vi "mclb_move_and_resize.vi"(8 "error in (no error)":errorcluster, 10 "Panel Resize.NewBnds":T3, 11 "mclb in":refnum<vi>) -> (0 "error out":errorcluster, 1 "MCLB.Bounds":T2, 2 "MCLB.Position":T1, 3 "mclb out":refnum<vi>, 4 "FP.Height":u32)   [LabVIEW 2017, in "rywindow.lvclass"]
uses:
  rywindow.lvclass
  <vilib>/Utility/miscctls.llb/LVRectTypeDef.ctl
  <vilib>/Utility/miscctls.llb/LVBoundsTypeDef.ctl
  <vilib>/Utility/miscctls.llb/LVPositionTypeDef.ctl
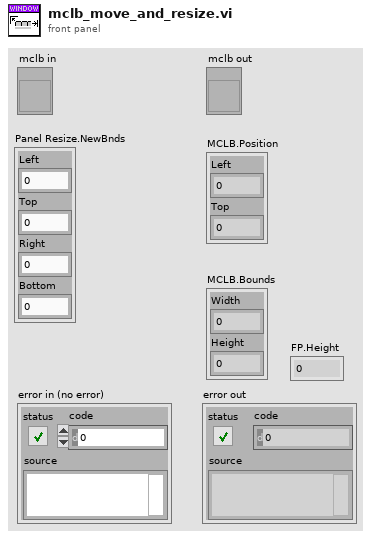
[diagram p1: front panel]
types:
  T1 = typedef "LVPositionTypeDef.ctl" = cluster{"Left":i32, "Top":i32}
  T2 = typedef "LVBoundsTypeDef.ctl" = cluster{"Width":u32, "Height":u32}
  T3 = typedef "LVRectTypeDef.ctl" = cluster{"Left":i16, "Top":i16, "Right":i16, "Bottom":i16}
  T4 = typedef "LVPointTypeDef.ctl" = cluster{"Horizontal":i16, "Vertical":i16}
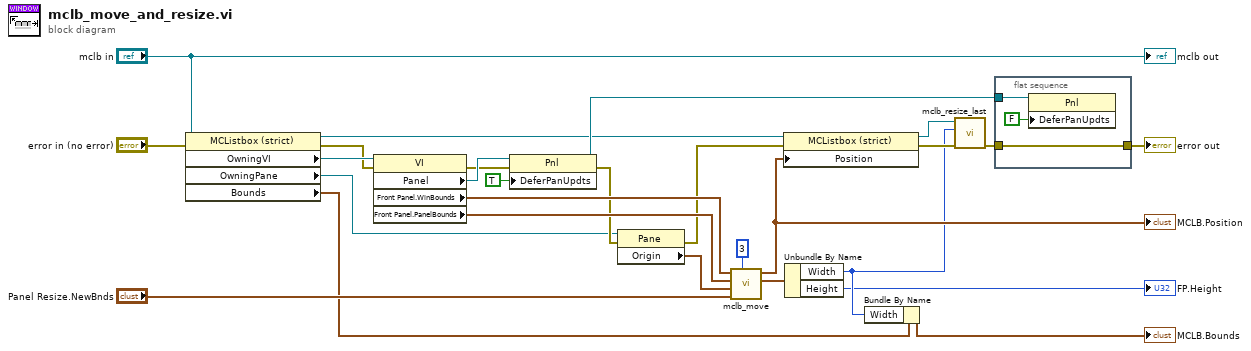
[diagram p0: block diagram]
diagram:
  n1 = property class="MCListbox (strict)"(reference="mclb in", error in="error in (no error)") -> (reference out=w6:refnum<vi>, error out=w8:errorcluster, "OwningVI"=w13:refnum<vi>, "OwningPane"=w9:refnum<vi>, "Bounds"=w4:T2)
  n2 = property class="VI"(reference=w13, error in=w8) -> (error out=w10:errorcluster, "Panel"=w25:refnum<vi>, "Front Panel.WinBounds"=w21:T3, "Front Panel.PanelBounds"=w22:T3)  [unwired: 1 out]
  n3 = property class="Pnl"(reference=w25, error in=w10, "DeferPanUpdts"=TRUE ("Defer Panel Updates")) -> (reference out=w26:refnum<vi>, error out=w14:errorcluster)
  n4 = property class="Pane"(reference=w9, error in=w14) -> (error out=w11:errorcluster, "Origin"=w20:T4)  [unwired: 1 out]
  n5 = call "mclb_move.vi"("remove bevel (3px)"=3, "Panel Resize.NewBnds"="Panel Resize.NewBnds", "FP.Origin"=w20, "FP.PanelBounds"=w22, "FP.WinBounds"=w21) -> ("bounds"=w12:T2, "pos"=w24:T1)  [unwired: 5 in]
  "MCLB.Position" <- w24
  n6 = property class="MCListbox (strict)"(reference=w6, error in=w11, "Position"=w24) -> (reference out=w19:refnum<vi>, error out=w18:errorcluster)
  n7 = Unbundle By Name(w12) -> ("Width"=w2:u32, "Height"=→"FP.Height":u32)
  n8 = Bundle By Name(cluster=w4, "Width"=w2) -> (→"MCLB.Bounds":T2)
  n9 = call "mclb_resize_last.vi"("error in (no error)"=w18, "FP.Width"=w2, "mclb in"=w19) -> ("error out"=w17:errorcluster)  [unwired: 7 in, 1 out]
  n10 = flat-sequence {
    tunnel: w26 -> [w29]
    tunnel: [w28] -> w16
    tunnel: w17 -> [w28]
    frame #0 {
      n11 = property class="Pnl"(reference=w29, "DeferPanUpdts"=FALSE ("Defer Panel Updates")) -> ()  [unwired: 1 in, 2 out]
    }
  }
  "error out" <- w16
  "mclb out" <- "mclb in"
